vi "test.vi"() -> ()   [LabVIEW 2013]
uses:
  message specification.ctl
  field descriptor.ctl
  quantity.ctl
  wire type.ctl
  protocol buffers encoder.lvlib
panel:
  out "logical AND":bool
  out "appended array":u8[](array[numeric])
  out "x = y?":bool[](array[boolean])
  out "byte array":u8[](array[numeric])
  out "submsg":variant
  out "error out":errorcluster
  out "message":variant
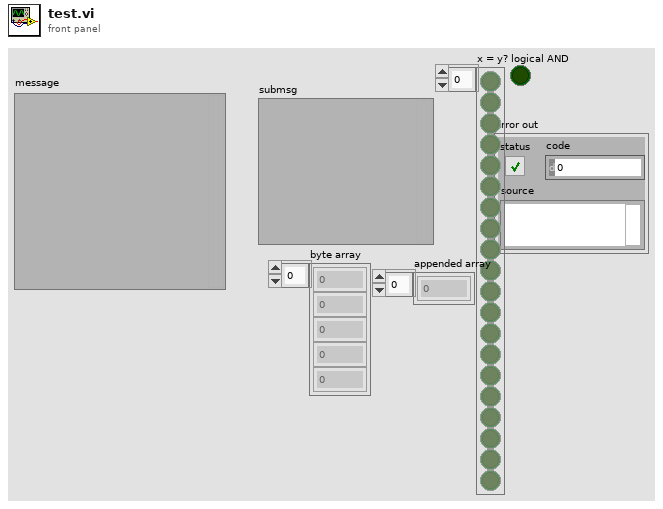
[diagram p1: front panel]
types:
  T1 = typedef "protocol buffers encoder.lvlib/wire type.ctl" = enum8{"Varint", "64 bit", "Length Delimited", "Start Group", "End Group", "32 bit"}
  T2 = typedef "protocol buffers encoder.lvlib/message specification.ctl" = cluster{"UID":u64, "name":string, "field descriptor":T3, "quantity":T4, "submessage":variant}
  T3 = typedef "protocol buffers encoder.lvlib/field descriptor.ctl" = enum16{"Unknown", "dbl", "sgl", "i64", "u64", "i32", "fixed64", "fixed32", "bool", "string", "group", "message", "bytes", "u32", "enum", "sfixed32", "sfixed64", "sint32", "sint64"}
  T4 = typedef "protocol buffers encoder.lvlib/quantity.ctl" = enum16{"required", "optional", "repeated", "repeated/packed"}
  T5 = typedef "protocol buffers encoder.lvlib/semiparse.ctl" = cluster{"wire type":T1, "field number":u64, "read index":i32, "length/data":u64}
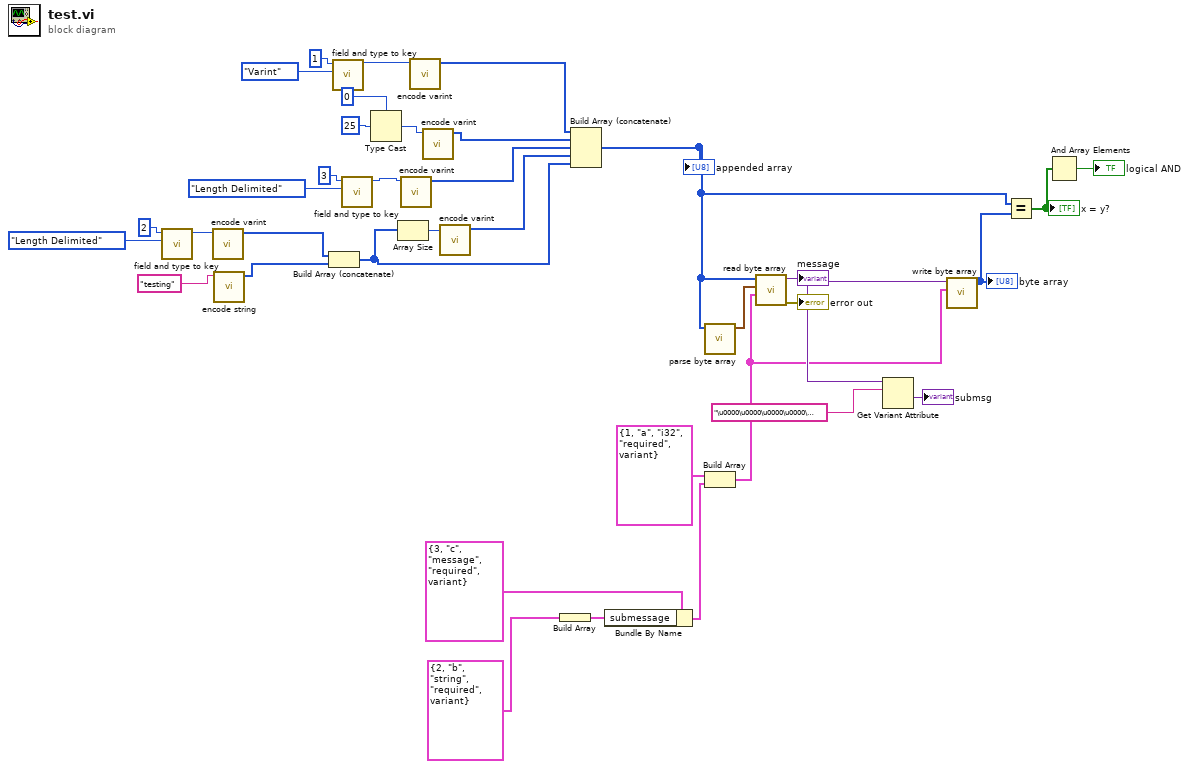
[diagram p0: block diagram]
diagram:
  n1 = call "field and type to key.vi"("wire type"=wire_type."Length Delimited", "field number"=u64 2) -> ("key"=w11:u64)  [unwired: 9 in]
  n2 = call "encode varint.vi"("value"=w11) -> ("byte array out"=w10:u8[])  [unwired: 10 in]
  n3 = call "encode string.vi"("String"="testing") -> ("byte array out"=w9:u8[])  [unwired: 10 in]
  n4 = Build Array (concatenate)(w10, w9) -> (w12:u8[])
  n5 = call "field and type to key.vi"("wire type"=wire_type."Varint", "field number"=u64 1) -> ("key"=w24:u64)  [unwired: 9 in]
  n6 = call "field and type to key.vi"("wire type"=wire_type."Length Delimited", "field number"=u64 3) -> ("key"=w16:u64)  [unwired: 9 in]
  n7 = Type Cast(type=u64 0 ("value"), x=25) -> (*(type *) &x=w21:u64)
  n8 = Array Size(array=w12) -> (size(s)=w14:i32)
  n9 = call "encode varint.vi"("value"=w16) -> ("byte array out"=w15:u8[])  [unwired: 10 in]
  n10 = call "encode varint.vi"("value"=w24) -> ("byte array out"=w19:u8[])  [unwired: 10 in]
  n11 = call "encode varint.vi"("value"=w21) -> ("byte array out"=w20:u8[])  [unwired: 10 in]
  n12 = call "encode varint.vi"("value"=w14) -> ("byte array out"=w13:u8[])  [unwired: 10 in]
  n13 = Build Array(T2 {"UID"=2, "name"="b", "field descriptor"=enum."string", "quantity"=enum."required", "submessage"=variant} ("message spec")) -> (w28:T2[])
  n14 = Build Array (concatenate)(w19, w20, w15, w13, w12) -> (w3:u8[])
  "appended array" <- w3
  n15 = Bundle By Name(cluster=T2 {"UID"=3, "name"="c", "field descriptor"=enum."message", "quantity"=enum."required", "submessage"=variant} ("message spec"), "submessage"=w28) -> (w33:T2)
  n16 = call "parse byte array.vi"("byte array"=w3) -> ("elements"=w36:T5[])  [unwired: 10 in]
  n17 = Build Array(T2 {"UID"=1, "name"="a", "field descriptor"=enum."i32", "quantity"=enum."required", "submessage"=variant} ("message spec"), w33) -> (w5:T2[])
  n18 = call "read byte array.vi"("specs"=w5, "elements"=w36, "byte array"=w3) -> ("error out"=→"error out":errorcluster, "message"=w6:variant)  [unwired: 7 in]
  "message" <- w6
  n19 = Get Variant Attribute(Variant=w6, name="\u0000\u0000\u0000\u0000\u0000\u0000\u0000\u0003") -> (value=→"submsg":variant)  [unwired: 2 in, 3 out]
  n20 = call "write byte array.vi"("specs"=w5, "message"=w6) -> ("byte array"=w4:u8[])  [unwired: 8 in, 1 out]
  "byte array" <- w4
  n21 = Equal?(x=w3, y=w4) -> (x = y?=w2:bool[])
  "x = y?" <- w2
  n22 = And Array Elements(Boolean array=w2) -> (logical AND=→"logical AND":bool)
